vi "心率报警.vi"(1 "心率":dbl, 2 "心率":refnum<vi>) -> (0 "心率情况":string)   [LabVIEW 2016]
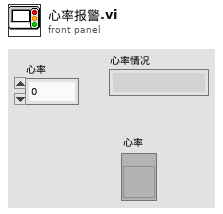
[diagram p1: front panel]
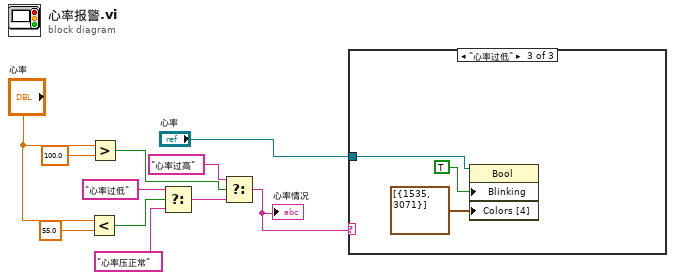
[diagram p0: block diagram]
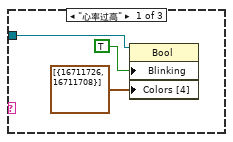
[diagram p2: hidden frame]
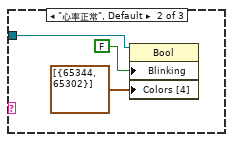
[diagram p3: hidden frame]
diagram:
  n1 = Less?(x="心率", y=55.0 ("心率下限")) -> (x < y?=w7:bool)
  n2 = Greater?(x="心率", y=100.0 ("心率上限")) -> (0:w10:bool)
  n3 = Select(t="心率过低", s=w7, f="心率压正常") -> (s? t:f=w9:string)
  n4 = Select(t="心率过高", s=w10, f=w9) -> (s? t:f=w3:string)
  "心率情况" <- w3
  n5 = case shown="\"心率过低\"" w3 {
    tunnel: "心率" -> [w14 w15 w18]
    frame "心率过高" {
      n6 = property class="Bool"(reference=w14, "Blinking"=TRUE ("闪烁"), "Colors [4]"=cluster{u32, u32}[] [{16711726, 16711708}] ("颜色[4]")) -> ()  [unwired: 1 in, 2 out]
    }
    frame "心率正常", Default {
      n7 = property class="Bool"(reference=w15, "Blinking"=FALSE ("闪烁"), "Colors [4]"=cluster{u32, u32}[] [{65344, 65302}] ("颜色[4]")) -> ()  [unwired: 1 in, 2 out]
    }
    frame "心率过低" {
      n8 = property class="Bool"(reference=w18, "Blinking"=TRUE ("闪烁"), "Colors [4]"=cluster{u32, u32}[] [{1535, 3071}] ("颜色[4]")) -> ()  [unwired: 1 in, 2 out]
    }
  }
